vi "Global_CMD_ACT_Data In.vi"() -> ()   [LabVIEW 2020, in "Cone_Stabber_ACT.lvlib"]
uses:
  ConeStabber/Cone_Stabber_ACT.lvlib
  Cluster_CMD_ACT_Data.ctl
  ConeStabber/ENUM_CMD_Cone_Stabber_Mode select.ctl
panel:
  in  "CMD_ACT_cone_stabber":T1
  # "The Names of the Data items in the Global Variable MUST describe who the Single Writer is\nFor Command Globals the Commander(CMD) represents Teleop or Autonomous or other command loop.\nThe naming convention for a Command Actuator Global is:   \n\nCMD_ACT_SubSystem_Data Name\n\nExample:\nCMD_ACT_Drive_Data\nCMD_ACT_Hopper_Eject Ball"
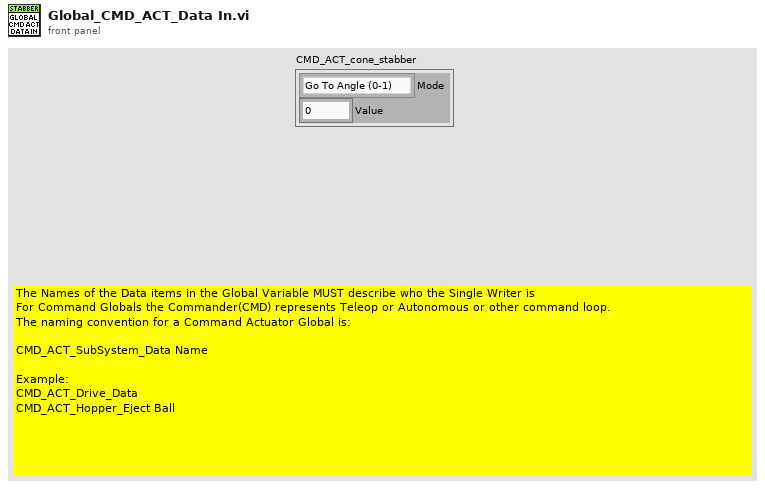
[diagram p1: front panel]
types:
  T1 = typedef "Cone_Stabber_ACT.lvlib/Cluster_CMD_ACT_Data.ctl" = cluster{"Mode":T2, "Value":dbl}
  T2 = typedef "Cone_Stabber_ACT.lvlib/ENUM_CMD_Cone_Stabber_Mode select.ctl" = enum16{"Go To Angle (0-1)", "Stop"}
diagram:
